vi "TagParser.vi"(11 "Channel Tag":string) -> (1 "Channel":i32, 2 "Module":i32, 3 "Chassis":i32)   [LabVIEW 2018, in "Controller (Host).lvlib"]
uses:
  Controller (Host).lvlib
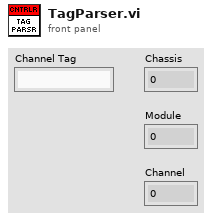
[diagram p1: front panel]
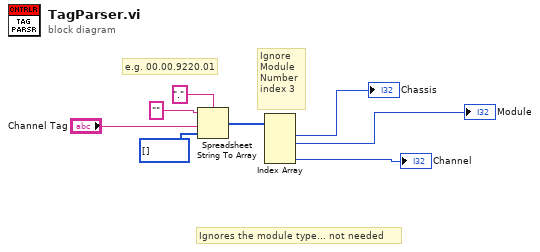
[diagram p0: block diagram]
diagram:
  # "Ignores the module type... not needed"
  # "e.g. 00.00.9220.01"
  # "Ignore\nModule\nNumber\nindex 3"
  n1 = Spreadsheet String To Array(delimiter (Tab)=".", format string="" ("spreadsheet string"), spreadsheet string="Channel Tag", array type (2D Dbl)=i32[] []) -> (array=w3:i32[])
  n2 = Index Array(array=w3) -> (element #1=→"Chassis":i32, element #2=→"Module":i32, element #4=→"Channel":i32)  [unwired: 4 in, 1 out]
